vi "GetDataTrProcMode.vi"(8 "错误输入（无错误）":errorcluster) -> (0 "错误输出":errorcluster, 3 "返回值":u8)   [LabVIEW 2018]
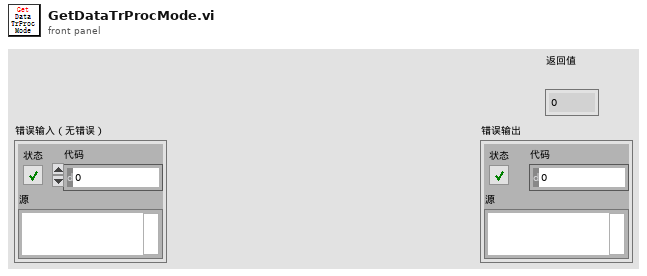
[diagram p1: front panel]
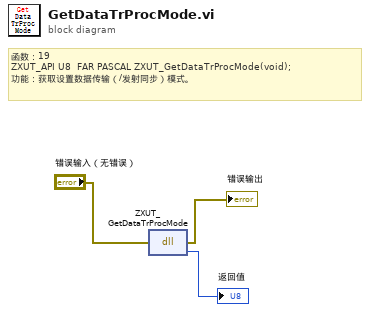
[diagram p0: block diagram]
diagram:
  # "函数：19\nZXUT_API U8\t\tFAR PASCAL ZXUT_GetDataTrProcMode(void);\n功能：获取设置数据传输（/发射同步）模式。"
  n1 = dll-call lib="PTH2Rabs E软件项目超声超声子VI函数VI\tTCG处理ZXUTConfigMgr.dll" fn="ZXUT_GetDataTrProcMode"(error in="错误输入（无错误）") -> (error out=→"错误输出":errorcluster, "返回值"=→"返回值":u8)  [unwired: 2 in, 1 out]
